vi "MeasureSystemOffset.vi"(8 "error in":errorcluster, 10 "Number of averages":u32=1, 11 "VISA resource name":refnum<visa-resource-name>) -> (0 "error out":errorcluster, 2 "Device offset from local / ms":dbl format="%.3f", 3 "VISA resource name out":refnum<visa-resource-name>)   [LabVIEW 2018, in "GP22_TDC_Arduinoed.lvlib"]
doc: "Use a basic version of NTP to calculate the offset of the device's system clock from the local PC's system clock."
uses:
  GP22_TDC_Arduinoed.lvlib
  <vilib>/Analysis/baseanly.llb/Mean (DBL).vi
  <vilib>/Analysis/NI_AALBase.lvlib
panel:
  out "Offset / ms":dbl(graph)
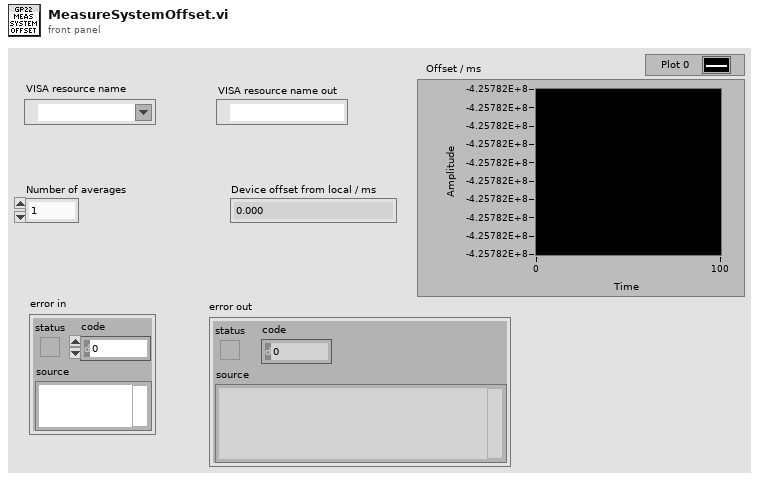
[diagram p1: front panel]
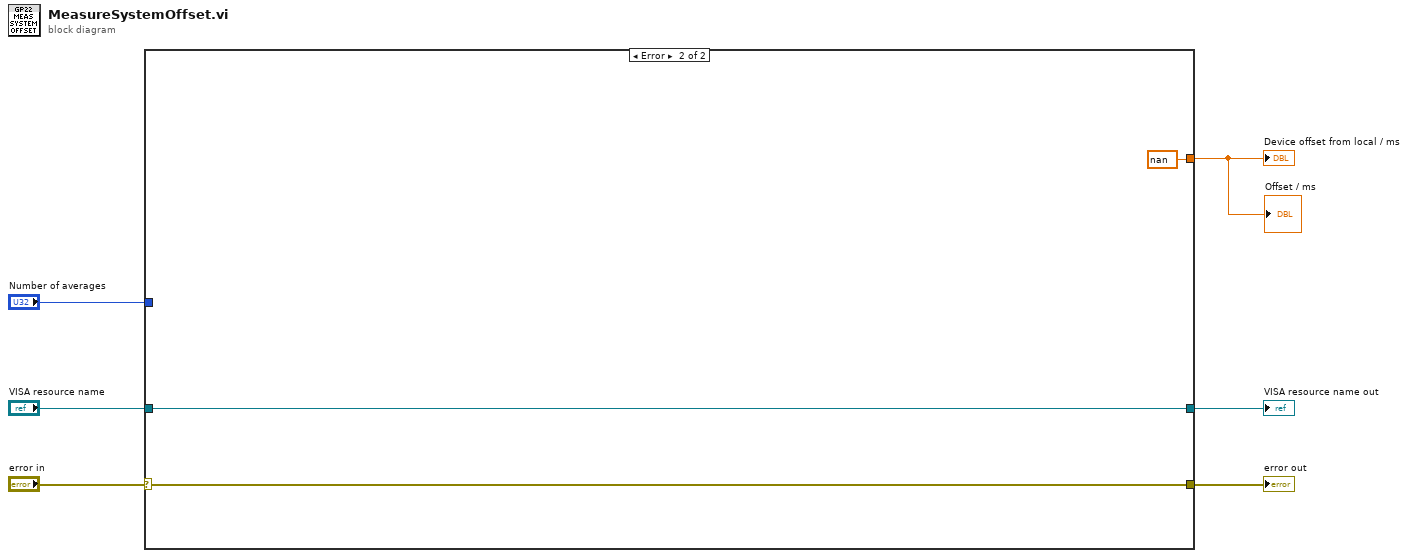
[diagram p0: block diagram]
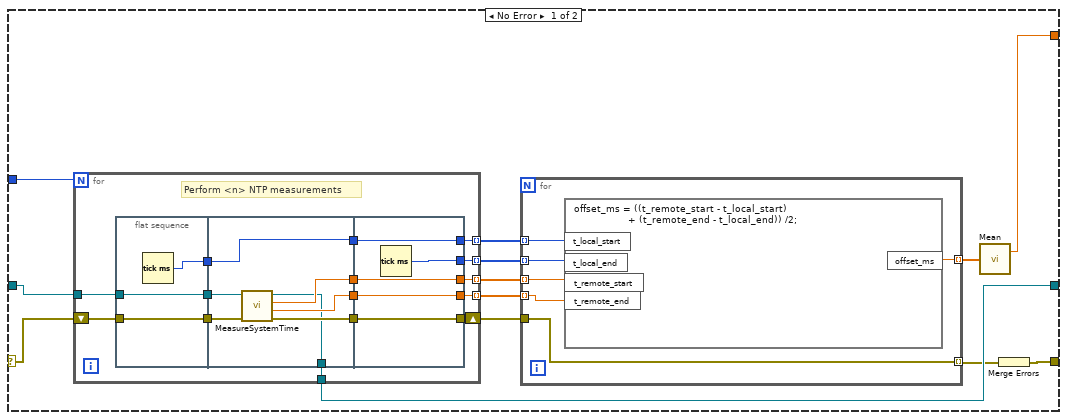
[diagram p2: hidden frame]
diagram:
  n1 = case shown="Error" "error in" {
    selector: "error in" -> [w18 w58]
    tunnel: [w11 w57] -> w6
    tunnel: "VISA resource name" -> [w19 w57]
    tunnel: [w10 w58] -> w3
    tunnel: "Number of averages" -> [w17 _]
    tunnel: [w7 nan] -> w1
    frame No Error {
      n2 = for {
        N: w17 -> [_]
        tunnel: w19 -> [w40]
        shift-right: [w38] -> w16
        shift-left: w18 -> [w39]
        tunnel: [w37] -> w13 mode=indexing
        tunnel: [w36] -> w12 mode=indexing
        tunnel: [w28] -> w15 mode=indexing
        tunnel: [w27] -> w14 mode=indexing
        tunnel: [w26] -> w11
        # "Perform <n> NTP measurements"
        n3 = flat-sequence {
          tunnel: w39 -> [w42]
          tunnel: w40 -> [w43]
          tunnel: [w43] -> w35
          tunnel: [w42] -> w34
          tunnel: [w41] -> w33
          tunnel: w35 -> [w50]
          tunnel: w34 -> [w49]
          tunnel: w33 -> [w45]
          tunnel: [w48] -> w32
          tunnel: [w47] -> w31
          tunnel: [w46] -> w30
          tunnel: [w45] -> w29
          tunnel: [w44] -> w26
          tunnel: [w52] -> w28
          tunnel: [w53] -> w36
          tunnel: [w54] -> w37
          tunnel: [w55] -> w38
          tunnel: w32 -> [w55]
          tunnel: w31 -> [w54]
          tunnel: w30 -> [w53]
          tunnel: w29 -> [w52]
          tunnel: [w51] -> w27
          frame #0 {
            n4 = Tick Count (ms)() -> (millisecond timer value=w41:u32)
          }
          frame #1 {
            n5 = call "MeasureSystemTime.vi"("error in"=w49, "VISA resource name"=w50) -> ("error out"=w48:errorcluster, "System time end"=w46:dbl, "System time start"=w47:dbl, "VISA resource name out"=w44:refnum<visa-resource-name>)  [unwired: 6 in]
          }
          frame #2 {
            n6 = Tick Count (ms)() -> (millisecond timer value=w51:u32)
          }
        }
      }
      n7 = for {
        tunnel: w16 -> [w21]
        tunnel: w15 -> [w25] mode=indexing
        tunnel: w14 -> [w24] mode=indexing
        tunnel: w13 -> [w23] mode=indexing
        tunnel: w12 -> [w22] mode=indexing
        tunnel: [w21] -> w9 mode=indexing
        tunnel: [w20] -> w8 mode=indexing
        n8 = formula code="offset_ms = ((t_remote_start - t_local_start) \n                  + (t_remote_end - t_local_end)) /2;"("t_local_start"=w25, "t_local_end"=w24, "t_remote_start"=w23, "t_remote_end"=w22) -> ("offset_ms"=w20:dbl)
      }
      n9 = call-poly <vilib>:"Mean.vi"("X"=w8) -> ("mean"=w7:dbl)  [unwired: 1 out]
      n10 = Merge Errors(w9) -> (w10:errorcluster)
    }
    frame Error {
    }
  }
  "VISA resource name out" <- w6
  "error out" <- w3
  "Device offset from local / ms" <- w1
  "Offset / ms" <- w1
